vi "探头窗口-4-网络版.vi"() -> ()   [LabVIEW 2017]
panel:
  in  "外部停止命令？":bool=TRUE
  out "引用-监测模式？":refnum<vi>
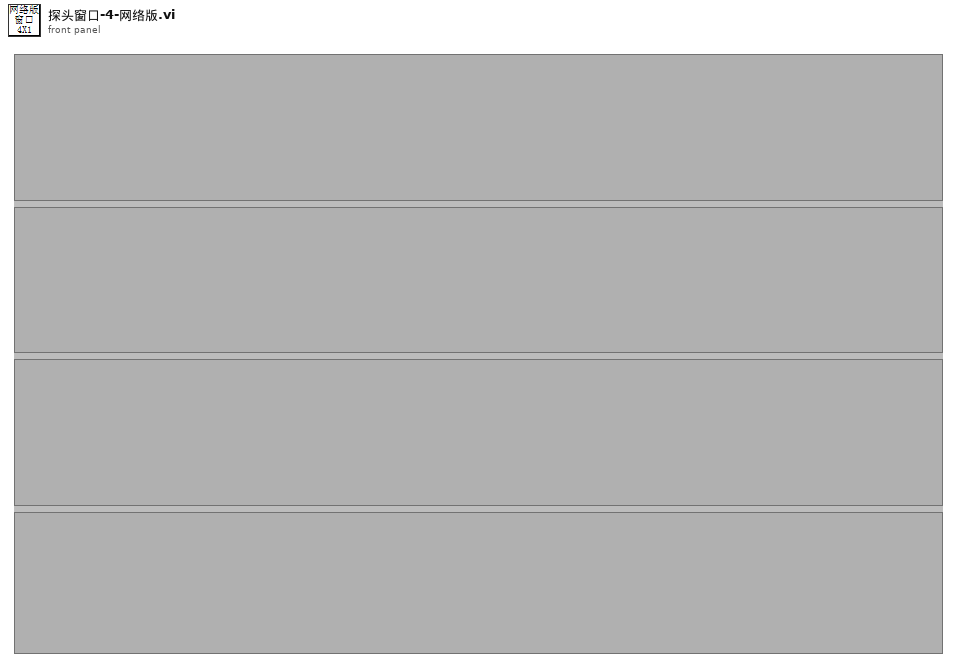
[diagram p1: front panel]
types:
  T1 = typedef "eventvkey.ctl" = enum16{"ASCII", "Enter", "Return", "Shift", "Ctrl", "Alt", "Cmd", "Opt", "Caps", "NumLock", "Clear", "Break", "Up", "Down", "Left", "Right", "Insert", "Delete", "Home", "End", "PageUp", "PageDown", "Escape", "Help", "Pause", "ScrollLock", "F1", "F2", "F3", "F4", "F5", "F6", "F7", "F8", "F9", "F10", "F11", "F12", "F13", "F14", "F15", "F16", "F17", "F18", "F19", "F20", "F21", "F22", "F23", "F24", "Play", "VolumeUp", "VolumeDown", "Mute", "Two Byte Char"}
  T2 = typedef "探头属性.ctl" = cluster{"探头地址与信息":T3, "测量值":T6, "限值":T7, "探头状态":T8, "累积记录":T9, "报警方式":T10}
  T3 = typedef "探测器信息.ctl" = cluster{"网络地址":string, "名称":string, "备注":string, "累积剂量":dbl, "累积限值":dbl, "硬件剂量率限值":T4, "剂量率限值1":dbl, "剂量率限值2":dbl, "报警方式":T5}
  T4 = typedef "探头剂量率限值选择.ctl" = enum16{"一级限值", "二级限值"}
  T5 = typedef "报警方式选择.ctl" = enum16{"常报警", "自动静音", "手动静音"}
  T6 = typedef "测量值.ctl" = cluster{"时间":timestamp, "数值":dbl}
  T7 = typedef "剂量率限值.ctl" = cluster{"限值1":dbl, "限值2":dbl, "探头限值":T4}
  T8 = typedef "探头状态.ctl" = enum16{"正常", "离线", "禁用", "一级报警", "二级报警", "累积报警"}
  T9 = typedef "单条累积记录.ctl" = cluster{"起始时间":timestamp, "结束时间":timestamp, "累积剂量":dbl}
  T10 = typedef "报警方式.ctl" = cluster{"报警方式":T5, "延迟计时":u16, "报警中？":bool}
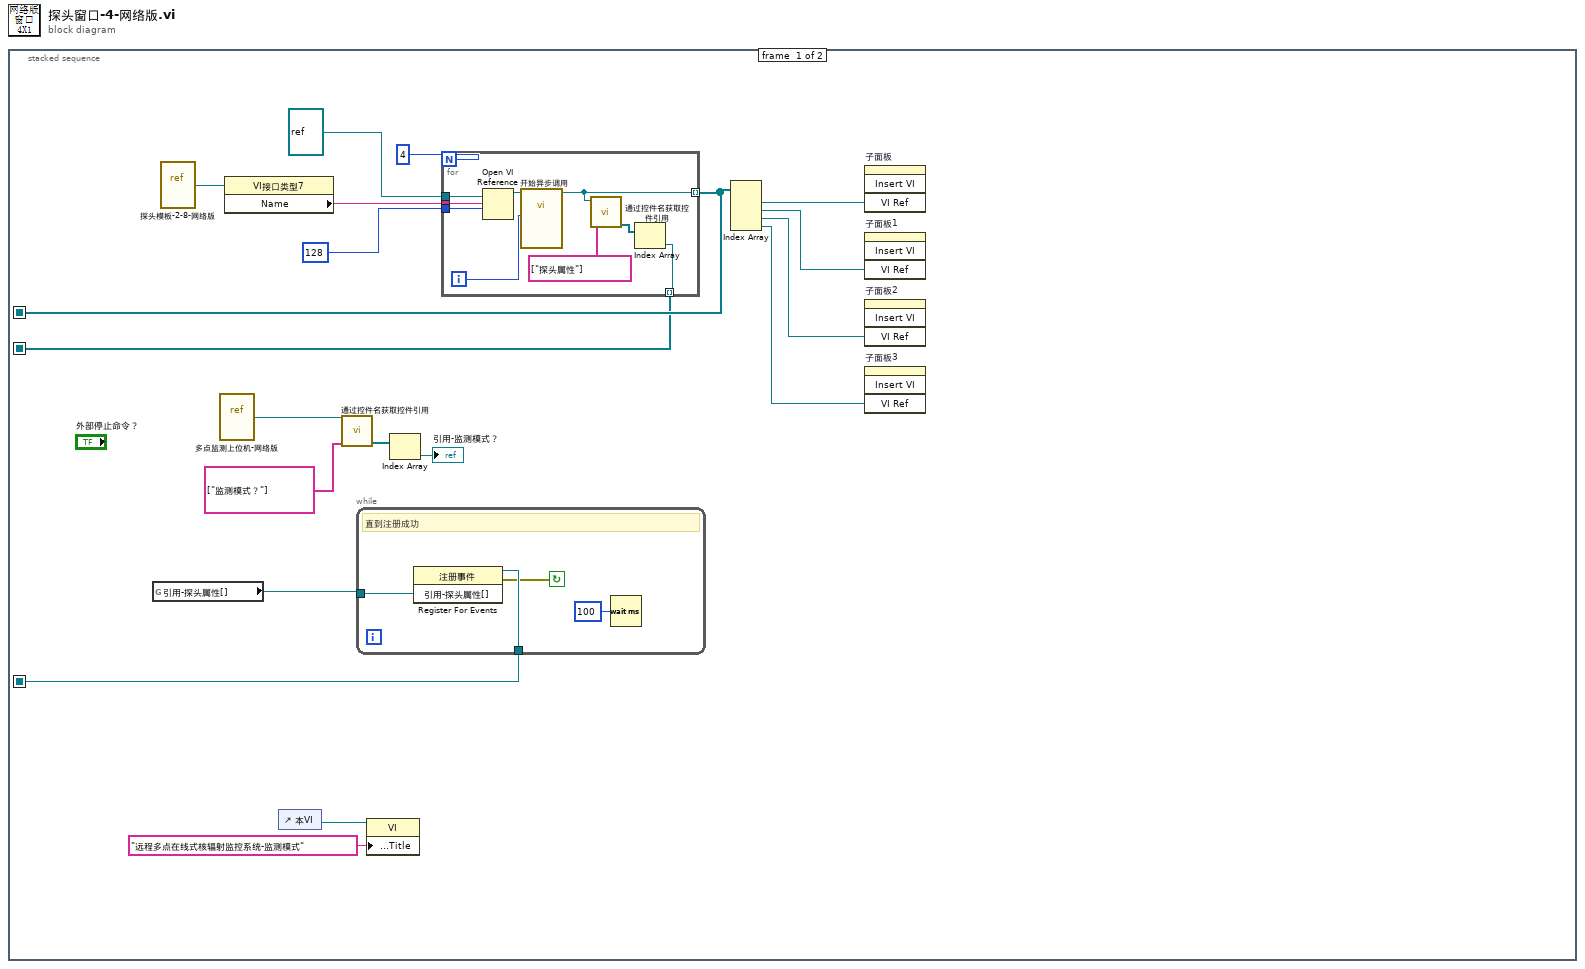
[diagram p0: block diagram]
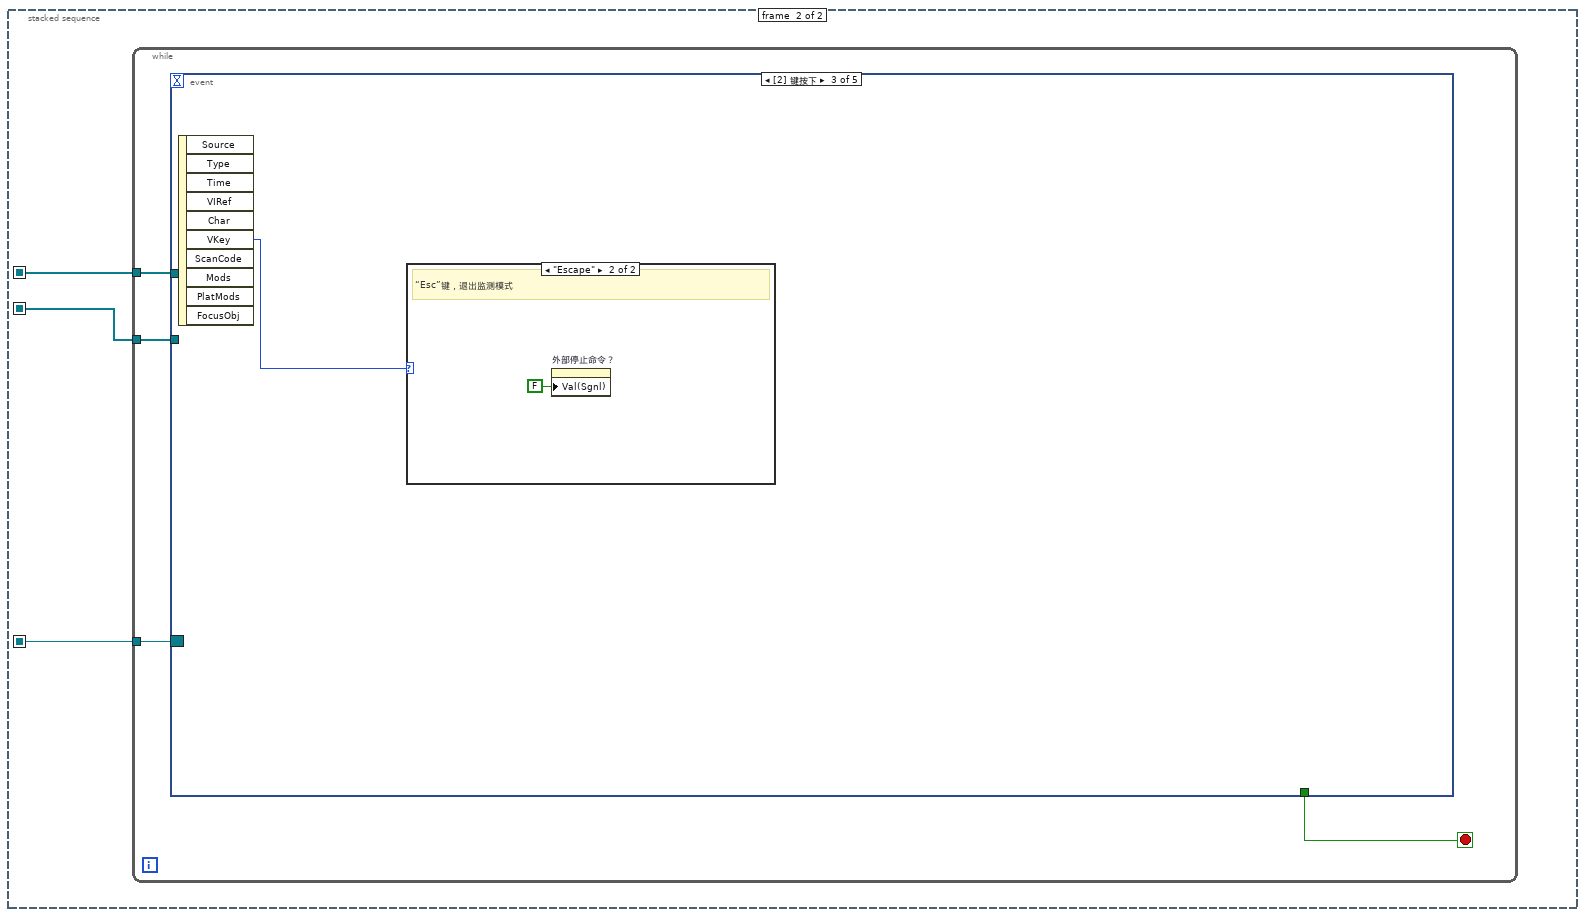
[diagram p2: hidden frame]
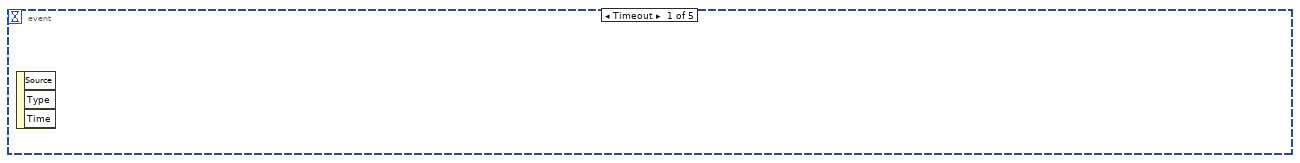
[diagram p3: hidden frame]
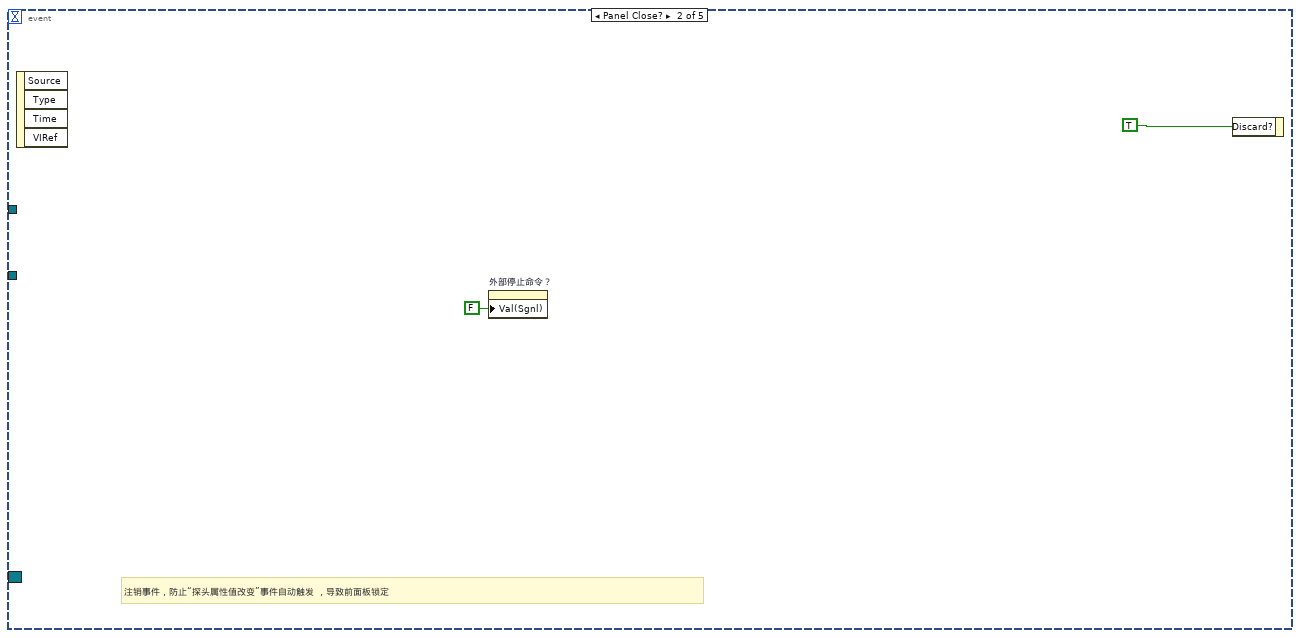
[diagram p4: hidden frame]
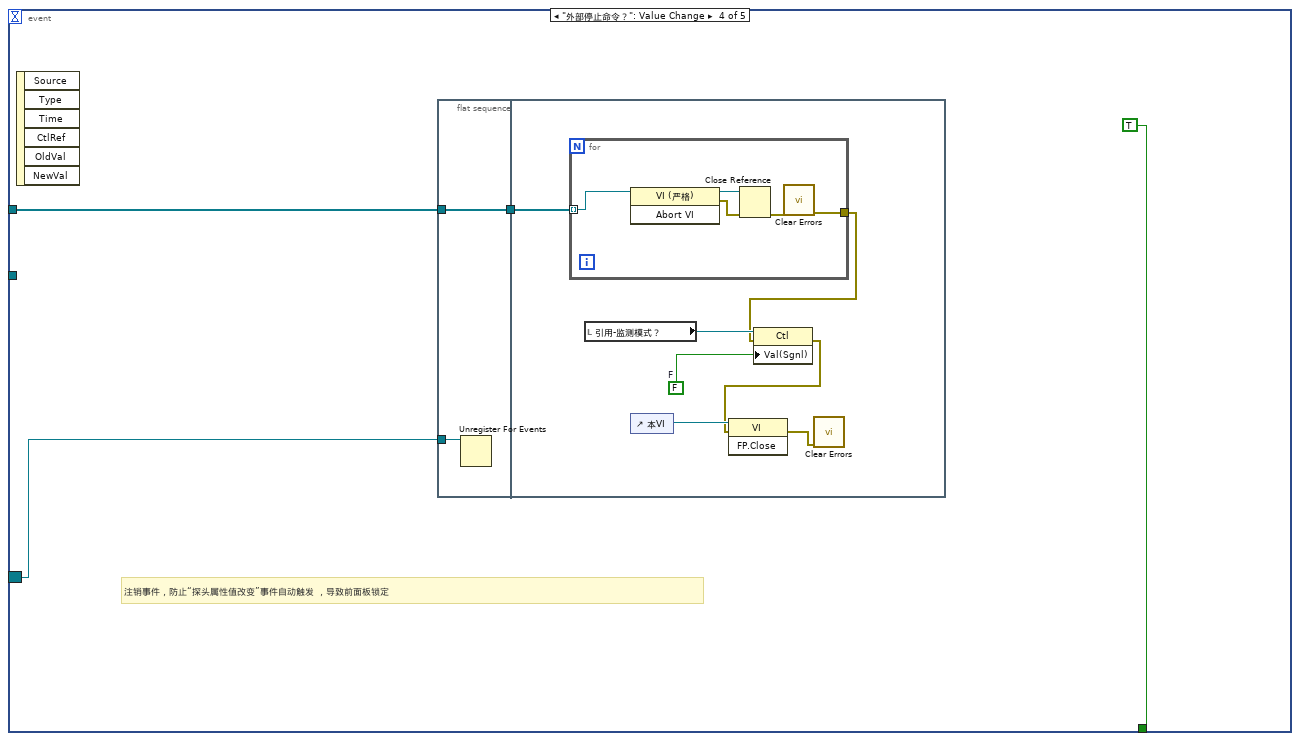
[diagram p6: hidden frame]
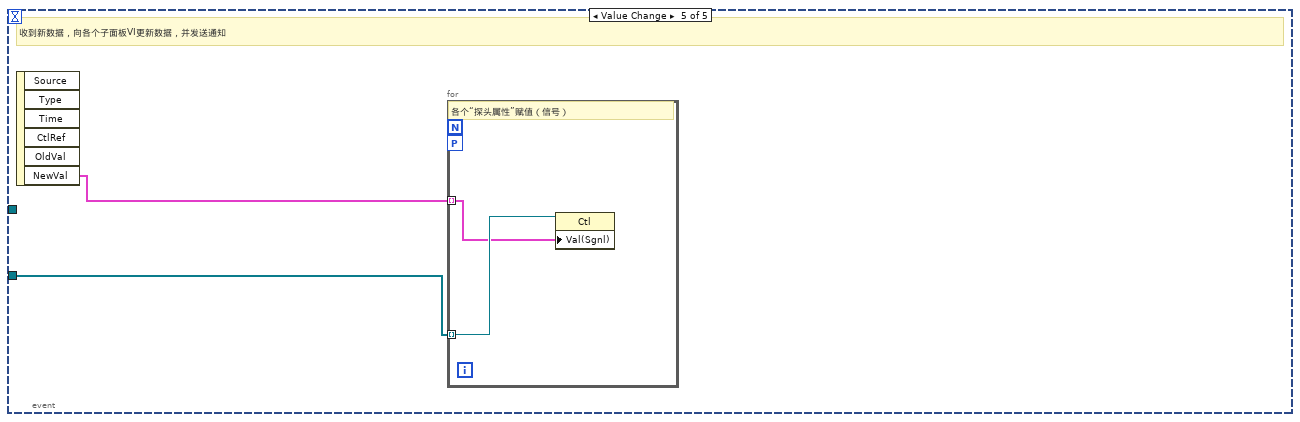
[diagram p7: hidden frame]
diagram:
  n1 = stacked-sequence {
    seq-local: [w15 _] -> [_ w35]
    seq-local: [w5 _] -> [_ w34]
    seq-local: [w1 _] -> [_ w33]
    frame #0 {
      n2 = global read "全局变量-35点监测.vi" "引用-探头属性[]"() -> (w2:refnum<vi>)
      n3 = vi-ref "探头模板-2-8-网络版.vi"() -> (w19:refnum<vi>)
      n4 = vi-ref "多点监测上位机-网络版.vi"() -> (w6:refnum<vi>)
      n5 = property class="VI接口类型7"(reference=w19) -> ("Name"=w18:string)  [unwired: 1 in, 2 out]
      n6 = control-ref of="本VI"() -> (w4:refnum<vi>)
      n7 = call "通过控件名获取控件引用.vi"("控件名数组"=string[] ["监测模式？"], "VI引用"=w6) -> ("控件引用输出"=w8:refnum<vi>[])  [unwired: 7 in, 2 out]
      n8 = while {
        tunnel: w2 -> [w23]
        tunnel: [w22] -> w1
        stop <- w21 continue-if-true
        # "直到注册成功"
        n9 = register-events(w23) -> (reference out=w22:refnum<event-registration>, error out=w21:errorcluster)  [unwired: 2 in]
        n10 = Wait (ms)(milliseconds to wait=u32 100 ("等待时间（毫秒）")) -> ()  [unwired: 1 out]
      }
      n11 = property class="VI"(reference=w4, "Front Panel.Title"="远程多点在线式核辐射监控系统-监测模式" ("前面板窗口:标题")) -> ()  [unwired: 1 in, 2 out]
      n12 = Index Array(array=w8) -> (element=→"引用-监测模式？":refnum<vi>)  [unwired: 1 in]
      n13 = for {
        N: 4 -> [_]
        tunnel: w18 -> [w32]
        tunnel: 128 ("选项") -> [w31]
        tunnel: refnum<vi> refnum ("类型说明符VI引用句柄（仅用于类型）") -> [w30]
        tunnel: [w25] -> w15 mode=indexing
        tunnel: [w26] -> w5 mode=indexing
        i -> [w24]
        n14 = Open VI Reference(type specifier VI Refnum (for type only)=w30, vi path=w32, options=w31) -> (vi reference=w27:refnum<vi>)  [unwired: 3 in, 1 out]
        n15 = call-by-ref "开始异步调用"(reference=w27, "探头序号"=w24) -> (reference out=w25:refnum<vi>)  [unwired: 12 in, 1 out]
        n16 = call "通过控件名获取控件引用.vi"("控件名数组"=string[] ["探头属性"], "VI引用"=w25) -> ("控件引用输出"=w29:refnum<vi>[])  [unwired: 7 in, 2 out]
        n17 = Index Array(array=w29) -> (element=w26:refnum<vi>)  [unwired: 1 in]
      }
      n18 = Index Array(array=w15) -> (element #1=w14:refnum<vi>, element #2=w13:refnum<vi>, element #3=w12:refnum<vi>, element #4=w11:refnum<vi>)  [unwired: 4 in]
      n19 = invoke on="子面板" class="子面板" method="Insert VI"("VI Ref"=w14) -> ()  [unwired: 3 in, 4 out]
      n20 = invoke on="子面板1" class="SubPnl" method="Insert VI"("VI Ref"=w13) -> ()  [unwired: 3 in, 4 out]
      n21 = invoke on="子面板2" class="SubPnl" method="Insert VI"("VI Ref"=w12) -> ()  [unwired: 3 in, 4 out]
      n22 = invoke on="子面板3" class="SubPnl" method="Insert VI"("VI Ref"=w11) -> ()  [unwired: 3 in, 4 out]
    }
    frame #1 {
      n23 = while {
        tunnel: w35 -> [w38]
        tunnel: w34 -> [w37]
        tunnel: w33 -> [w36]
        stop <- w39 stop-if-true
        n24 = event shown="[2] 键按下" {
          selector: w36 -> [_ _ _ w44 _]
          dyn-events: _ -> [_ _ _ _ _]
          timeout: _ -> [_ _ _ _ _]
          tunnel: [_ _ _ TRUE ("放弃？") _] -> w39
          tunnel: w38 -> [_ _ _ w46 _]
          tunnel: w37 -> [_ _ _ _ w62]
          event Timeout {
            n25 = event-data() -> ()  [unwired: 1 in, 3 out]
          }
          event Panel Close? {
            # "注销事件，防止“探头属性值改变”事件自动触发 ，导致前面板锁定"
            n26 = event-data() -> ()  [unwired: 1 in, 4 out]
            n27 = property on="外部停止命令？" class="Bool (严格)"("Val(Sgnl)"=FALSE ("值(信号)")) -> ()  [unwired: 2 in, 2 out]
            n28 = event-data("Discard?"=TRUE ("放弃？")) -> ()  [unwired: 1 in, 1 out]
          }
          event Key Down {
            n29 = event-data() -> ("VKey"=w42:T1)  [unwired: 1 in, 9 out]
            n30 = case shown="\"Escape\"" w42 {
              frame "ASCII", Default {
              }
              frame "Escape" {
                # "“Esc”键，退出监测模式"
                n31 = property on="外部停止命令？" class="Bool (严格)"("Val(Sgnl)"=FALSE ("值(信号)")) -> ()  [unwired: 2 in, 2 out]
              }
            }
          }
          event "外部停止命令？": Value Change {
            # "注销事件，防止“探头属性值改变”事件自动触发 ，导致前面板锁定"
            n32 = event-data() -> ()  [unwired: 1 in, 6 out]
            n33 = flat-sequence {
              tunnel: w46 -> [w49]
              tunnel: [w49] -> w45
              tunnel: w44 -> [w48]
              tunnel: w45 -> [w56]
              frame #0 {
                n34 = Unregister For Events(event registration refnum=w48) -> ()  [unwired: 1 in, 1 out]
              }
              frame #1 {
                w55 = FALSE  # F
                n35 = for {
                  tunnel: w56 -> [w61] mode=indexing
                  tunnel: [w57] -> w51
                  n36 = invoke class="VI (严格)" method="Abort VI"(reference=w61) -> (reference out=w59:refnum<vi>, error out=w60:errorcluster)  [unwired: 2 in, 1 out]
                  n37 = Close Reference(reference=w59, error in (no error)=w60) -> (error out=w58:errorcluster)
                  n38 = call <vilib>:"Clear Errors.vi"("error in (no error)"=w58) -> ("error out"=w57:errorcluster)  [unwired: 5 in, 1 out]
                }
                n39 = local read "引用-监测模式？"() -> (w54:refnum<vi>)
                n40 = control-ref of="本VI"() -> (w53:refnum<vi>)
                n41 = property class="Ctl"(reference=w54, error in=w51, "Val(Sgnl)"=w55) -> (error out=w52:errorcluster)  [unwired: 1 out]
                n42 = invoke class="VI" method="FP.Close"(reference=w53, error in=w52) -> (error out=w50:errorcluster)  [unwired: 1 in, 2 out]
                n43 = call <vilib>:"Clear Errors.vi"("error in (no error)"=w50) -> ()  [unwired: 5 in, 2 out]
              }
            }
          }
          event Value Change {
            # "收到新数据，向各个子面板VI更新数据，并发送通知"
            n44 = event-data() -> ("NewVal"=w63:T2[])  [unwired: 1 in, 5 out]
            n45 = for {
              workers-P: _ -> [_]
              tunnel: w62 -> [w65] mode=indexing
              tunnel: w63 -> [w64] mode=indexing
              # "各个“探头属性”赋值（信号）"
              n46 = property class="Ctl"(reference=w65, "Val(Sgnl)"=w64) -> ()  [unwired: 1 in, 2 out]
            }
          }
        }
      }
    }
  }
